vi "Communication - Serial Number (FGV).vi"(7 "Action":T1, 8 "error in (no error)":errorcluster, 10 "Device Name":string[](array[string]), 11 "S/N":string[](array[string])) -> (0 "error out":errorcluster, 2 "Device Name Out":string[](array[string]), 3 "S/N Out":string[](array[string]))   [LabVIEW 2019]
uses:
  Controls/FGV States.ctl
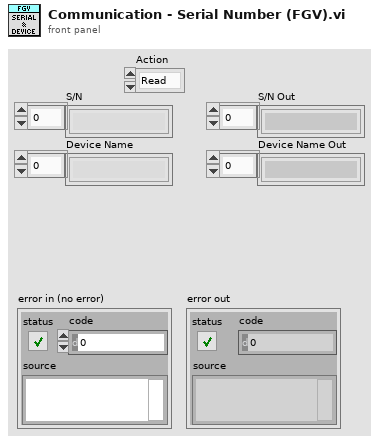
[diagram p1: front panel]
types:
  T1 = typedef "FGV States.ctl" = enum16{"Read", "Write"}
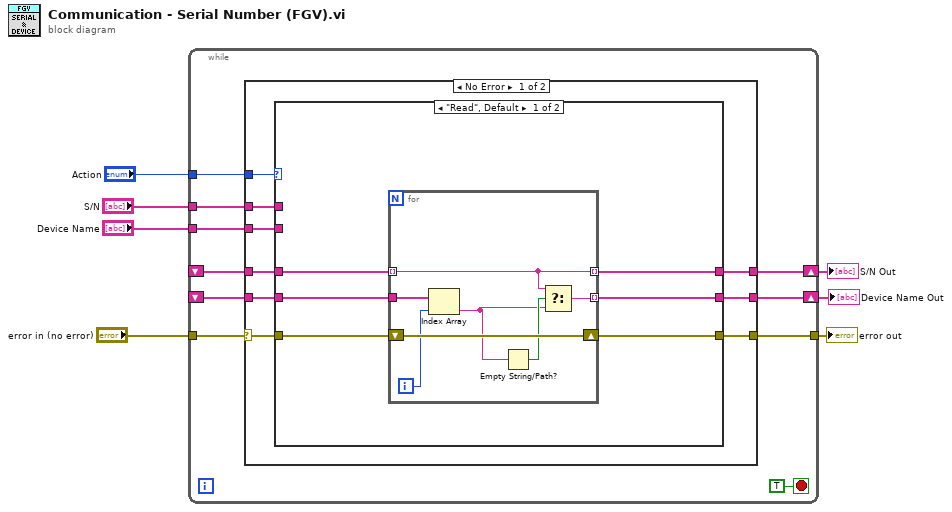
[diagram p0: block diagram]
diagram:
  n1 = while {
    tunnel: "Action" -> [w17]
    tunnel: "S/N" -> [w15]
    shift-right: [w16] -> w5
    shift-left: _ -> [w14]
    tunnel: "error in (no error)" -> [w12]
    tunnel: [w11] -> w3
    tunnel: "Device Name" -> [w10]
    shift-right: [w9] -> w1
    shift-left: _ -> [w8]
    stop <- TRUE stop-if-true
    n2 = case shown="No Error" w12 {
      selector: w12 -> [w21 w44]
      tunnel: w17 -> [w26 _]
      tunnel: [w25 w45] -> w16
      tunnel: w15 -> [w24 _]
      tunnel: w14 -> [w23 w45]
      tunnel: [w22 w44] -> w11
      tunnel: w10 -> [w20 _]
      tunnel: [w19 w43] -> w9
      tunnel: w8 -> [w18 w43]
      frame No Error {
        n3 = case shown="\"Read\", Default" w26 {
          tunnel: [w30 w42] -> w25
          tunnel: w24 -> [_ w42]
          tunnel: w23 -> [w29 _]
          tunnel: [w32 w41] -> w22
          tunnel: w21 -> [w31 w41]
          tunnel: w20 -> [_ w40]
          tunnel: [w27 w40] -> w19
          tunnel: w18 -> [w28 _]
          frame "Read", Default {
            n4 = for {
              shift-right: [w39] -> w32
              shift-left: w31 -> [w39]
              tunnel: [w34] -> w30 mode=indexing
              tunnel: w29 -> [w34] mode=indexing
              tunnel: w28 -> [w38]
              tunnel: [w33] -> w27 mode=indexing
              i -> [w37]
              n5 = Index Array(array=w38, index=w37) -> (element=w35:string)
              n6 = Empty String/Path?(string/path=w35) -> (empty?=w36:bool)
              n7 = Select(t=w34, s=w36, f=w35) -> (s? t:f=w33:string)
            }
          }
          frame "Write" {
          }
        }
      }
      frame Error {
      }
    }
  }
  "S/N Out" <- w5
  "error out" <- w3
  "Device Name Out" <- w1
